vi "DAQ Analog Trigger.vi"(0 "Channels":tag[](array[tag])=["Dev1/ai1", "Dev1/ai2"], 3 "trigger edge":i32(ring)=10171 items=["Rising"=10280, "Falling"=10171], 4 "trigger level":dbl=2.5, 7 "number of samples":i32=100, 9 "rate":dbl=1000.0, 11 "error in":errorcluster, 13 "timeout (s)":dbl=10.0 format="%0.2f") -> (8 "data":dynamicdata(waveform), 14 "Timed Out":bool, 15 "error out":errorcluster)   [LabVIEW 2014]
doc: "This vi grabs an array of voltage waveforms in response to the defined trigger condition\n\nMatt Strader\nPaul K Dixon\nPhysics 350\nCSUSB Physics"
uses:
  <vilib>/DAQmx/read.llb/DAQmx Read.vi
  <vilib>/DAQmx/read.llb/DAQmx Read (Analog 1D Wfm NChan NSamp).vi
  <vilib>/DAQmx/miscellaneous.llb/DAQmx Fill In Error Info.vi
  <vilib>/DAQmx/configure/trigger.llb/DAQmx Trigger.vi
  <vilib>/DAQmx/configure/trigger.llb/DAQmx Start Trigger (Analog Edge).vi
  <vilib>/DAQmx/configure/timing.llb/DAQmx Timing (Sample Clock).vi
  <vilib>/DAQmx/create/channels.llb/DAQmx Create Channel (AI-Voltage-Basic).vi
  <vilib>/DAQmx/create/channels.llb/DAQmx Create Channel (TEDS-AI-Voltage-Basic).vi
panel:
  in  "stop (T)":bool=TRUE
  out "task out":refnum<k21>
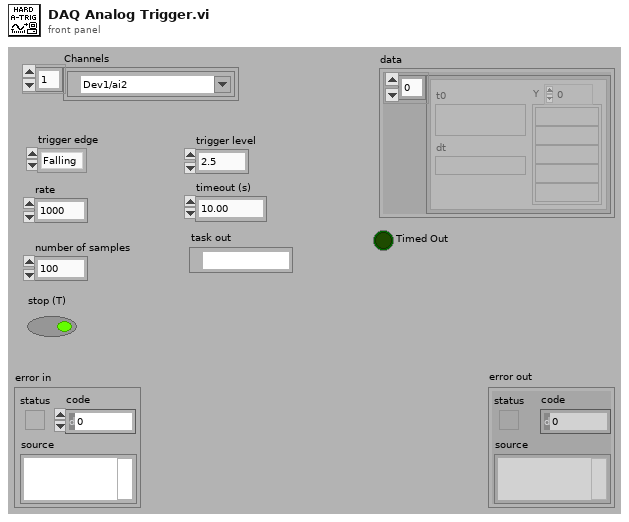
[diagram p1: front panel]
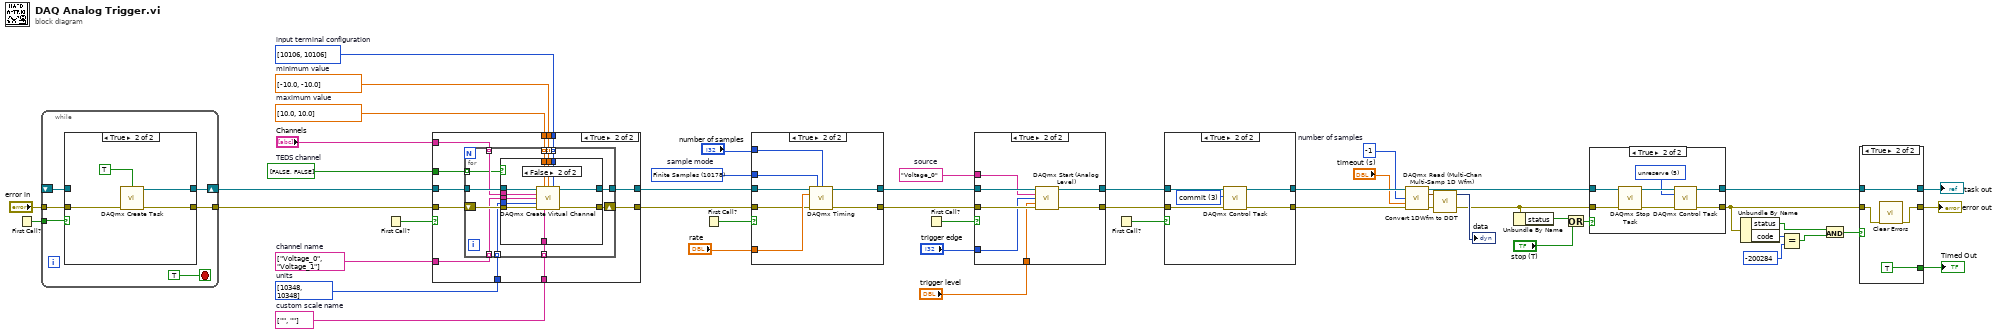
[diagram p0: block diagram]
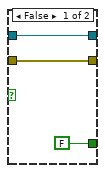
[diagram p2: hidden frame]
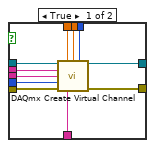
[diagram p8: hidden frame]
diagram:
  w20 = -1  # number of samples
  w27 = "Voltage_0"  # source
  w31 = 10178 items=["Finite Samples"=10178, "Continuous Samples"=10123, "Hardware Timed Single Point"=12522]  # sample mode
  w37 = bool[] [FALSE, FALSE]  # TEDS channel
  w38 = string[] ["", ""]  # custom scale name
  w39 = i32[] [10348, 10348] items=["Volts"=10348, "From TEDS"=12516, "From Custom Scale"=10065]  # units
  w40 = string[] ["Voltage_0", "Voltage_1"]  # channel name
  w41 = dbl[] [10.0, 10.0]  # maximum value
  w42 = dbl[] [-10.0, -10.0]  # minimum value
  w43 = i32[] [10106, 10106] items=["default"=-1, "RSE"=10083, "NRSE"=10078, "Differential"=10106, "Pseudodifferential"=12529]  # input terminal configuration
  n1 = First Call?() -> (First Call?: T/F=w49:bool)
  n2 = while {
    shift-right: [w54] -> w45
    shift-left: _ -> [w53]
    tunnel: w49 -> [w55]
    tunnel: [w52] -> w48
    tunnel: "error in" -> [w51]
    stop <- TRUE stop-if-true
    n3 = case shown="True" w55 {
      tunnel: [w57 w61] -> w54
      tunnel: w53 -> [w57 _]
      tunnel: [w56 w60] -> w52
      tunnel: w51 -> [w56 w58]
      frame False {
      }
      frame True {
        n4 = call <vilib>:"DAQmx Create Task.vi"("auto cleanup"=TRUE, "error in"=w58) -> ("task out"=w61:refnum<k21>, "error out"=w60:errorcluster)  [unwired: 3 in, 9 out]
      }
    }
  }
  n5 = First Call?() -> (First Call?: T/F=w46:bool)
  n6 = case shown="True" w46 {
    tunnel: [w63 w73] -> w35
    tunnel: w45 -> [w63 w75]
    tunnel: [w62 w72] -> w44
    tunnel: w48 -> [w62 w74]
    tunnel: w43 -> [_ w71]
    tunnel: w42 -> [_ w70]
    tunnel: w41 -> [_ w69]
    tunnel: "Channels" -> [_ w68]
    tunnel: w40 -> [_ w67]
    tunnel: w39 -> [_ w66]
    tunnel: w38 -> [_ w65]
    tunnel: w37 -> [_ w64]
    frame False {
    }
    frame True {
      n7 = for {
        tunnel: w75 -> [w87]
        tunnel: [w85] -> w73
        tunnel: w71 -> [w83] mode=indexing
        tunnel: w70 -> [w82] mode=indexing
        tunnel: w69 -> [w81] mode=indexing
        tunnel: w68 -> [w80] mode=indexing
        tunnel: w67 -> [w79] mode=indexing
        tunnel: w66 -> [w78] mode=indexing
        tunnel: w65 -> [w77] mode=indexing
        shift-right: [w84] -> w72
        shift-left: w74 -> [w86]
        tunnel: w64 -> [w76] mode=indexing
        n8 = case shown="False" w76 {
          tunnel: w87 -> [w98 w109]
          tunnel: w86 -> [w97 w108]
          tunnel: [w96 w107] -> w85
          tunnel: [w95 w106] -> w84
          tunnel: w83 -> [w94 w105]
          tunnel: w82 -> [w93 w104]
          tunnel: w81 -> [w92 w103]
          tunnel: w80 -> [w91 w102]
          tunnel: w79 -> [w90 w101]
          tunnel: w78 -> [w89 w100]
          tunnel: w77 -> [w88 w99]
          frame True {
            n9 = call-poly <vilib>:"DAQmx Create Virtual Channel.vi"("task in"=w98, "maximum value"=w92, "minimum value"=w93, "input terminal configuration"=w94, "physical channels"=w91, "name to assign"=w90, "units"=w89, "error in"=w97, "custom scale name"=w88) -> ("task out"=w96:refnum<k21>, "error out"=w95:errorcluster)  [unwired: 5 out]
          }
          frame False {
            n10 = call-poly <vilib>:"DAQmx Create Virtual Channel.vi"("task in"=w109, "maximum value"=w103, "minimum value"=w104, "input terminal configuration"=w105, "physical channels"=w102, "name to assign"=w101, "units"=w100, "error in"=w108, "custom scale name"=w99) -> ("task out"=w107:refnum<k21>, "error out"=w106:errorcluster)  [unwired: 5 out]
          }
        }
      }
    }
  }
  n11 = First Call?() -> (First Call?: T/F=w36:bool)
  n12 = case shown="True" w36 {
    tunnel: [w111 w113] -> w29
    tunnel: w35 -> [w111 w116]
    tunnel: [w110 w112] -> w34
    tunnel: w44 -> [w110 w114]
    tunnel: "number of samples" -> [_ w118]
    tunnel: w31 -> [_ w117]
    tunnel: "rate" -> [_ w115]
    frame False {
    }
    frame True {
      n13 = call-poly <vilib>:"DAQmx Timing.vi"("task/channels in"=w116, "sample mode"=w117, "samples per channel"=w118, "rate"=w115, "error in"=w114) -> ("task out"=w113:refnum<k21>, "error out"=w112:errorcluster)  [unwired: 2 in, 7 out]
    }
  }
  n14 = First Call?() -> (First Call?: T/F=w30:bool)
  n15 = case shown="True" w30 {
    tunnel: [w120 w125] -> w23
    tunnel: w29 -> [w120 w127]
    tunnel: [w119 w124] -> w28
    tunnel: w34 -> [w119 w126]
    tunnel: w27 -> [_ w123]
    tunnel: "trigger edge" -> [_ w122]
    tunnel: "trigger level" -> [_ w121]
    frame False {
    }
    frame True {
      n16 = call-poly "DAQmx Start (Analog Level).vi"("task/channels in"=w127, "source"=w123, "slope"=w122, "level"=w121, "error in"=w126) -> ("task out"=w125:refnum<k21>, "error out"=w124:errorcluster)  [unwired: 9 out]
    }
  }
  n17 = First Call?() -> (First Call?: T/F=w24:bool)
  n18 = case shown="True" w24 {
    tunnel: [w129 w133] -> w21
    tunnel: w23 -> [w129 w134]
    tunnel: [w128 w131] -> w22
    tunnel: w28 -> [w128 w132]
    frame False {
    }
    frame True {
      w130 = 3 items=["verify"=2, "reserve"=4, "commit"=3, "unreserve"=5, "abort"=6] ("action")
      n19 = call <vilib>:"DAQmx Control Task.vi"("task/channels in"=w134, "action"=w130, "error in"=w132) -> ("task out"=w133:refnum<k21>, "error out"=w131:errorcluster)  [unwired: 11 out]
    }
  }
  n20 = call-poly "DAQmx Read (Multi-Chan Multi-Samp 1D Wfm).vi"("task/channels in"=w21, "number of samples per channel"=w20, "timeout"="timeout (s)", "error in"=w22) -> ("task out"=w4:refnum<k21>, "data"=w19:waveform(dbl)[], "error out"=w3:errorcluster)  [unwired: 9 out]
  n21 = call <vilib>:"Convert 1DWfm to DDT.vi"("Array of Waveforms"=w19) -> ("Dynamic Data Type"=→"data":dynamicdata)  [unwired: 3 out]
  n22 = Unbundle By Name(w3) -> ("status"=w17:bool)
  n23 = Or(x=w17, y="stop (T)") -> (x .or. y?=w15:bool)
  n24 = case shown="True" w15 {
    tunnel: [w135 w138] -> w5
    tunnel: [w136 w141] -> w2
    tunnel: w3 -> [w136 w143]
    tunnel: w4 -> [w135 w137]
    frame False {
    }
    frame True {
      w139 = 5 items=["verify"=2, "reserve"=4, "commit"=3, "unreserve"=5, "abort"=6] ("action")
      n25 = call <vilib>:"DAQmx Stop Task.vi"("task/channels in"=w137, "error in"=w143) -> ("task out"=w140:refnum<k21>, "error out"=w142:errorcluster)  [unwired: 12 out]
      n26 = call <vilib>:"DAQmx Control Task.vi"("task/channels in"=w140, "action"=w139, "error in"=w142) -> ("task out"=w138:refnum<k21>, "error out"=w141:errorcluster)  [unwired: 11 out]
    }
  }
  n27 = Unbundle By Name(w2) -> ("status"=w8:bool, "code"=w7:i32)
  n28 = Equal?(x=w7, y=-200284) -> (x = y?=w9:bool)
  n29 = And(x=w8, y=w9) -> (x .and. y?=w10:bool)
  n30 = case shown="True" w10 {
    tunnel: [w144 w149] -> w11
    tunnel: [w146 w150] -> w12
    tunnel: w5 -> [w146 w150]
    tunnel: [FALSE TRUE] -> w1
    tunnel: w2 -> [w144 w147]
    frame False {
    }
    frame True {
      n31 = call <vilib>:"Clear Errors.vi"("error in (no error)"=w147) -> ("error out"=w149:errorcluster)  [unwired: 1 in, 5 out]
    }
  }
  "task out" <- w12
  "error out" <- w11
  "Timed Out" <- w1
